vi "DeferPanelUpdate.vi"(8 "error in (no error)":errorcluster, 10 "Defer Panel Updates":bool, 11 "GObjectRefIn":refnum<vi>) -> (0 "error out":errorcluster)   [LabVIEW 2013, in "VariableManagerAPI.lvlib"]
doc: "When you set this property to TRUE, LabVIEW redraws any front panel objects with pending changes then defers all new requests for front panel updates. For example, controls and indicators do not redraw when their properties or values change. If the operating system requests a redraw, such as if the window is no longer behind another window, LabVIEW redraws the front panel with the current properties instead of the original properties. If FALSE, LabVIEW immediately redraws the changed elements of the front panel.\n\nSetting this property to TRUE can improve the execution speed and memory usage of a VI."
uses:
  VariableManagerAPI.lvlib
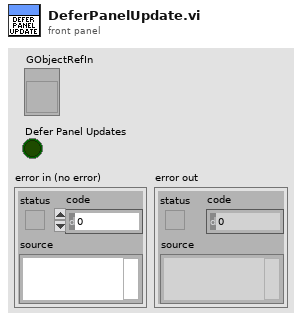
[diagram p1: front panel]
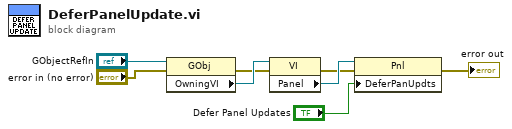
[diagram p0: block diagram]
diagram:
  n1 = property class="GObj"(reference="GObjectRefIn", error in="error in (no error)") -> (error out=w5:errorcluster, "OwningVI"=w6:refnum<vi>)  [unwired: 1 out]
  n2 = property class="VI"(reference=w6, error in=w5) -> (error out=w3:errorcluster, "Panel"=w4:refnum<vi>)  [unwired: 1 out]
  n3 = property class="Pnl"(reference=w4, error in=w3, "DeferPanUpdts"="Defer Panel Updates") -> (error out=→"error out":errorcluster)  [unwired: 1 out]
